vi "B7_65_Check_Init_STB_4_Error.vi"(4 "Error Code":T6=5490, 6 "Driver Name":T7="B1_28", 8 "error in":T8, 11 "DriverConnect in":T1={"InterfaceType"=enum."VISA", "OpenedSession"="", "InterfaceSettings"={"Interface"=enum."RS232", "EOS 4 read"=enum."LF (\\n)", "EOS 4 write"=enum."LF (\\n)", "TMO, ms"=10000, "Sett"=variant(cluster{"Baud Rate":u32, "Data Bits":u16, "Parity":u16, "Stop Bits":u16, "Flow Control":u16, "Eho":bool} {"Baud Rate"=75, "Data Bits"=0, "Parity"=0, "Stop Bits"=0, "Flow Control"=0, "Eho"=FALSE})}}) -> (0 "error out":T8, 3 "DriverConnect out":T1={"InterfaceType"=enum."VISA", "OpenedSession"="", "InterfaceSettings"={"Interface"=enum."RS232", "EOS 4 read"=enum."LF (\\n)", "EOS 4 write"=enum."LF (\\n)", "TMO, ms"=10000, "Sett"=variant(cluster{"Baud Rate":u32, "Data Bits":u16, "Parity":u16, "Stop Bits":u16, "Flow Control":u16, "Eho":bool} {"Baud Rate"=75, "Data Bits"=0, "Parity"=0, "Stop Bits"=0, "Flow Control"=0, "Eho"=FALSE})}})   [LabVIEW 2018]
uses:
  MOKO_LabViewLibrary/MokoLowLevel/MokoLowLovelControl/MLLC_Error.ctl
  MOKO_LabViewLibrary/MokoLowLevel/MokoLowLovelControl/MLLC_DriverName.ctl
  MOKO_LabViewLibrary/MokoLowLevel/MokoLowLovelControl/MLLC_ErrorCode.ctl
  MOKO_LabViewLibrary/MokoLowLevel/MokoLowLovelControl/MLLC_ConnectCluster.ctl
  MOKO_LabViewLibrary/MokoLowLevel/MokoLowLovelControl/MLLC_InterfaceType.ctl
  MOKO_LabViewLibrary/MokoLowLevel/MokoLowLovelControl/MLLC_OpenedSession.ctl
  MOKO_LabViewLibrary/MokoLowLevel/MokoLowLovelControl/MLLC_InterfaceSettings.ctl
  MOKO_LabViewLibrary/MokoLowLevel/MokoLowLovelControl/MLLC_InterfaceKind.ctl
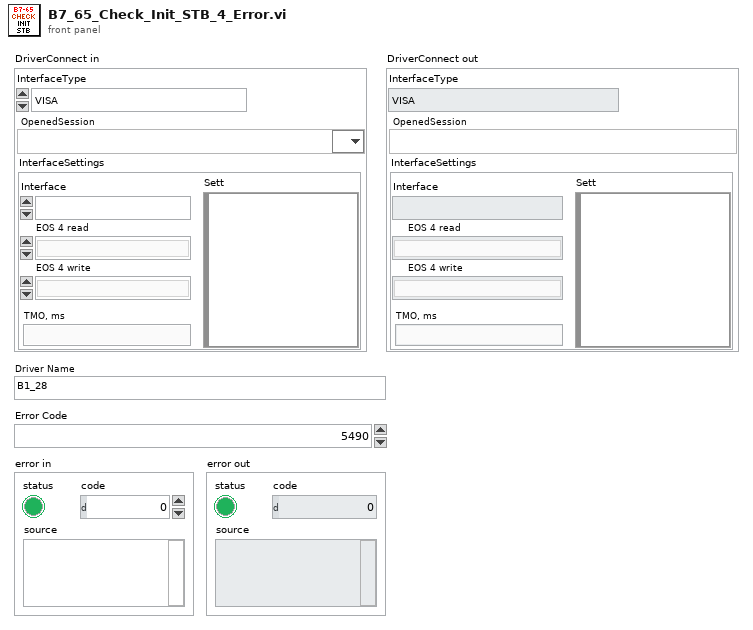
[diagram p1: front panel]
types:
  T1 = typedef "MLLC_ConnectCluster.ctl" = cluster{"InterfaceType":T2, "OpenedSession":T3, "InterfaceSettings":T4}
  T2 = typedef "MLLC_InterfaceType.ctl" = enum16{"VISA", "Prologix USB-GPIB"}
  T3 = typedef "MLLC_OpenedSession.ctl" = refnum<visa-resource-name>
  T4 = typedef "MLLC_InterfaceSettings.ctl" = cluster{"Interface":T5, "EOS 4 read":enum16{"Default (=EOS 4 write)", "CR (\\r)", "LF (\\n)", "None"}, "EOS 4 write":enum16{"CR+LF (\\r\\n)", "CR (\\r)", "LF (\\n)", "None"}, "TMO, ms":i32, "Sett":variant}
  T5 = typedef "MLLC_InterfaceKind.ctl" = enum16{"RS232", "GPIB", "USB", "Ethernet", "another"}
  T6 = typedef "MLLC_ErrorCode.ctl" = u32
  T7 = typedef "MLLC_DriverName.ctl" = string
  T8 = typedef "MLLC_Error.ctl" = errorcluster
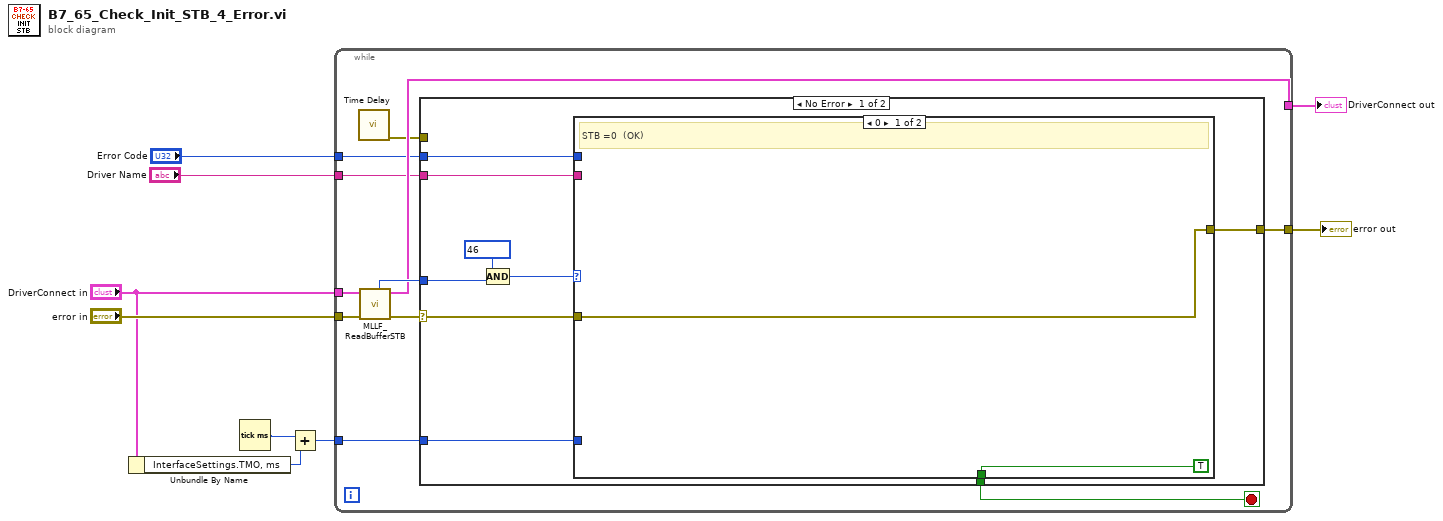
[diagram p0: block diagram]
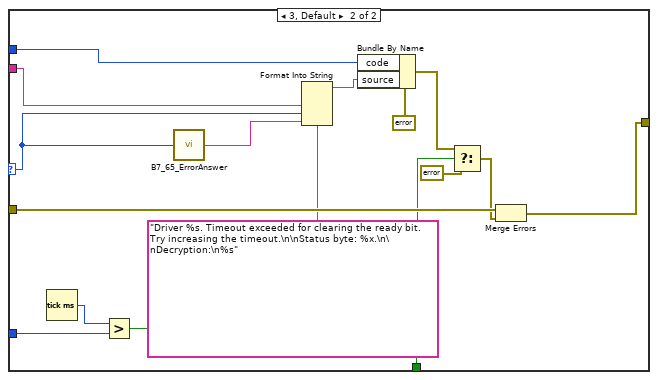
[diagram p2: hidden frame]
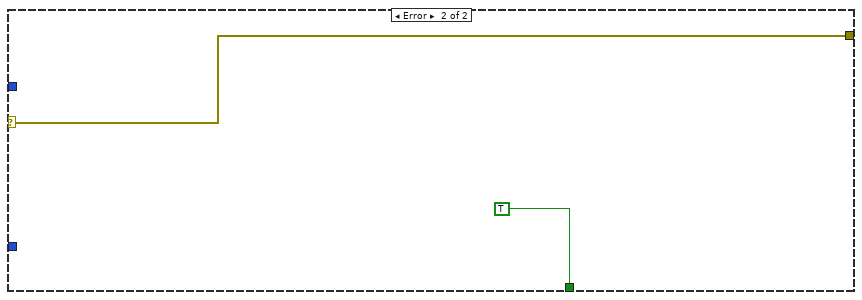
[diagram p3: hidden frame]
diagram:
  n1 = Unbundle By Name("DriverConnect in") -> ("InterfaceSettings.TMO, ms"=w7:i32)
  n2 = Tick Count (ms)() -> (millisecond timer value=w6:u32)
  n3 = Add(x=w6, y=w7) -> (x+y=w5:u32)
  n4 = while {
    tunnel: [w20] -> w9
    tunnel: "error in" -> [w19]
    tunnel: [w16] -> w1
    tunnel: w5 -> [w14]
    tunnel: "Error Code" -> [w13]
    tunnel: "Driver Name" -> [w12]
    tunnel: "DriverConnect in" -> [w11]
    stop <- w15 stop-if-true
    n5 = call "Time Delay"() -> ("error out"=w10:errorcluster)  [unwired: 11 in]
    n6 = call "MLLF_ReadBufferSTB.vi"("Error In"=w19, "DriverConnect in"=w11) -> ("Error Out"=w17:errorcluster, "DriverConnect out"=w16:T1, "Status byte"=w18:u16)  [unwired: 7 in]
    n7 = case shown="No Error" w17 {
      selector: w17 -> [w28 w48]
      tunnel: [w29 w48] -> w20
      tunnel: w18 -> [w22 _]
      tunnel: [w27 TRUE] -> w15
      tunnel: w14 -> [w26 _]
      tunnel: w13 -> [w25 _]
      tunnel: w12 -> [w24 _]
      tunnel: w10 -> [_ _]
      frame No Error {
        n8 = Compound Arithmetic op=AND(u8 46 ("status"), w22) -> (w21:u16)
        n9 = case shown="0" w21 {
          selector: w21 -> [_ w36]
          tunnel: [w31 w41] -> w29
          tunnel: w28 -> [w31 w42]
          tunnel: [TRUE w39] -> w27
          tunnel: w26 -> [_ w45]
          tunnel: w25 -> [_ w38]
          tunnel: w24 -> [_ w34]
          frame 0 {
            # "STB =0  (OK)"
          }
          frame 3, Default {
            n10 = Tick Count (ms)() -> (millisecond timer value=w46:u32)
            n11 = Greater?(x=w46, y=w45) -> (0:w39:bool)
            n12 = call "B7_65_ErrorAnswer.vi"("input"=w36) -> ("Error answer string"=w35:string)  [unwired: 4 in]
            n13 = Format Into String(format string="Driver %s. Timeout exceeded for clearing the ready bit. Try increasing the timeout.\n\nStatus byte: %x.\n\nDecryption:\n%s", w34, w36, w35) -> (resulting string=w32:string)  [unwired: 2 in, 1 out]
            n14 = Bundle By Name(cluster=errorcluster {"status"=TRUE, "code"=5100, "source"="B1-28. Timeout."} ("error in"), "code"=w38, "source"=w32) -> (w43:errorcluster)
            n15 = Select(t=w43, s=w39, f=errorcluster {"status"=FALSE, "code"=0, "source"=""} ("error in")) -> (s? t:f=w40:errorcluster)
            n16 = Merge Errors(w42, w40) -> (w41:errorcluster)
          }
        }
      }
      frame Error {
      }
    }
  }
  "error out" <- w9
  "DriverConnect out" <- w1
